vi "init_data_out.vi"(8 "error in (no error)":errorcluster, 11 "output channel":refnum<k21>) -> (0 "error out":errorcluster, 3 "task out":refnum<k24>)   [LabVIEW 2015]
uses:
  C:/Program Files/National Instruments/LabVIEW 2015/vi.lib/ULx/ULx_LV.dll
  <vilib>/ULx/Create Channel.llb/ULx Create Channel (AO-Voltage-Basic).vi
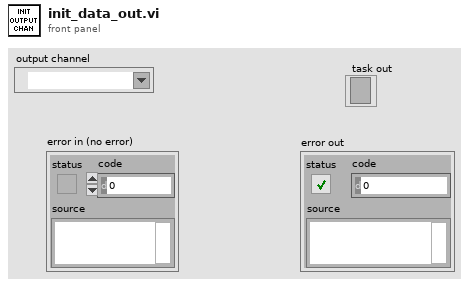
[diagram p1: front panel]
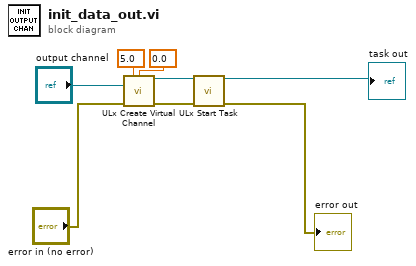
[diagram p0: block diagram]
diagram:
  n1 = call-poly <vilib>:"ULx Create Virtual Channel.vi"("maximum value"=5.0 ("Maximum Value"), "minimum value"=0.0 ("Minimum Value"), "physical channels"="output channel", "error in"="error in (no error)") -> ("task out"=w5:refnum<k24>, "error out"=w6:errorcluster)  [unwired: 10 in]
  n2 = call <vilib>:"ULx Start Task.vi"("task in"=w5, "error in"=w6) -> ("task out"=→"task out":refnum<k24>, "error out"=→"error out":errorcluster)  [unwired: 12 in]
